vi "Write to Hardware.vi"(8 "error in":errorcluster, 9 "trigger values":dbl[](array[numeric]), 10 "values":dbl[](array[numeric]), 11 "tx execution unit":refnum<class "Tx Execution Unit.lvclass">) -> (0 "error out":errorcluster, 1 "trigger values out":dbl[](array[numeric]), 2 "values out":dbl[](array[numeric]), 3 "tx execution unit out":refnum<class "Tx Execution Unit.lvclass">)   [LabVIEW 2020, in "AIM MIL-STD-1553 Engine.lvlib" / "Implementation.lvlib" / "Tx Execution Unit.lvclass"]
uses:
  Tx Execution Unit.lvclass
  C:/dev/git/niveristand-aim-milStd1553-custom-device/Source/Custom Device Support/Engine/Implementation/Execution Unit/Execution Unit.lvclass
  Execution Unit/Execution Unit.lvclass/Execution Unit.ctl
  Tx Execution Unit.lvclass/Tx Execution Unit.ctl
  Shared/Message Definition.ctl
  Shared/Message Type.ctl
  Shared/Terminal Endpoint.ctl
  Shared/Address.ctl
  Shared/Parameter Definition.ctl
  Execution Unit/Read Module Reference.vi
  Read Transmitted Messages.vi
  Hardware API/AIM MIL-STD-1553 Hardware API.lvlib
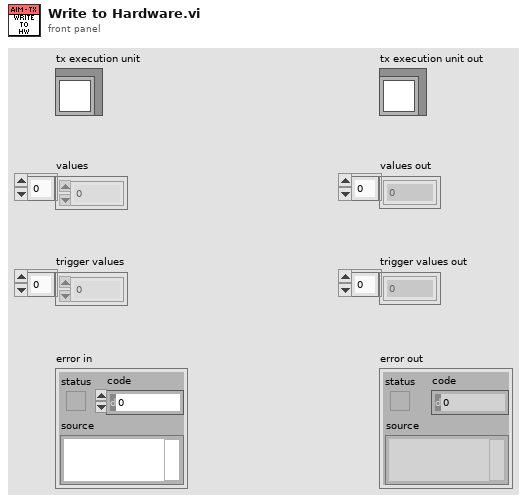
[diagram p1: front panel]
types:
  T1 = typedef "AIM MIL-STD-1553 Hardware API.lvlib/Module Reference.ctl" = u32
  T2 = typedef "AIM MIL-STD-1553 Engine.lvlib/Custom Device.lvlib/Compiled Message.ctl" = cluster{"Message Section Handle":T3, "First Parameter Index":i32, "Parameter Channel Handles":T3[], "Direction":T4, "Parameters":T5[], "Receiving RT Address":u8, "Receiving RT Sub-address":u8, "Transmitting RT Address":u8, "Transmitting RT Sub-address":u8, "Word Count":u8, "Buffer Type":enum16{"unknown", "BC Message Buffer", "RT Message Buffer"}, "Buffer ID":u16, "Terminal Type":enum16{"Bus Controller", "Remote Terminal"}, "Timestamp Enabled":bool, "Timestamp Channel Handle":T3}
  T3 = typedef "Custom Device API.lvlib/Custom Device Item Ref.ctl" = u64
  T4 = typedef "Direction.ctl" = enum16{"Rx", "Tx"}
  T5 = typedef "Parameter Definition.ctl" = cluster{"start index":i32, "size (bits)":i32, "encoding":enum16{"BNR", "BCD", "Discrete"}, "signed":bool, "multiplier":dbl, "offset":dbl}
  T6 = typedef "Message Definition.ctl" = cluster{"name":string, "message type":T7, "endpoint Tx":T8, "endpoint Rx":T8, "create timestamp channel":bool, "mode code":u16, "number of words":u16, "parameters":cluster{"name":string, "default value":dbl, "unit":string, "parameter definition":T5}[]}
  T7 = typedef "Message Type.ctl" = string
  T8 = typedef "Terminal Endpoint.ctl" = cluster{"terminal address":T9, "subaddress":T9}
  T9 = typedef "Address.ctl" = u16
  T10 = cluster{"name":string, "default value":dbl, "unit":string, "parameter definition":T5}
  T11 = enum16{"unknown", "BC Message Buffer", "RT Message Buffer"}
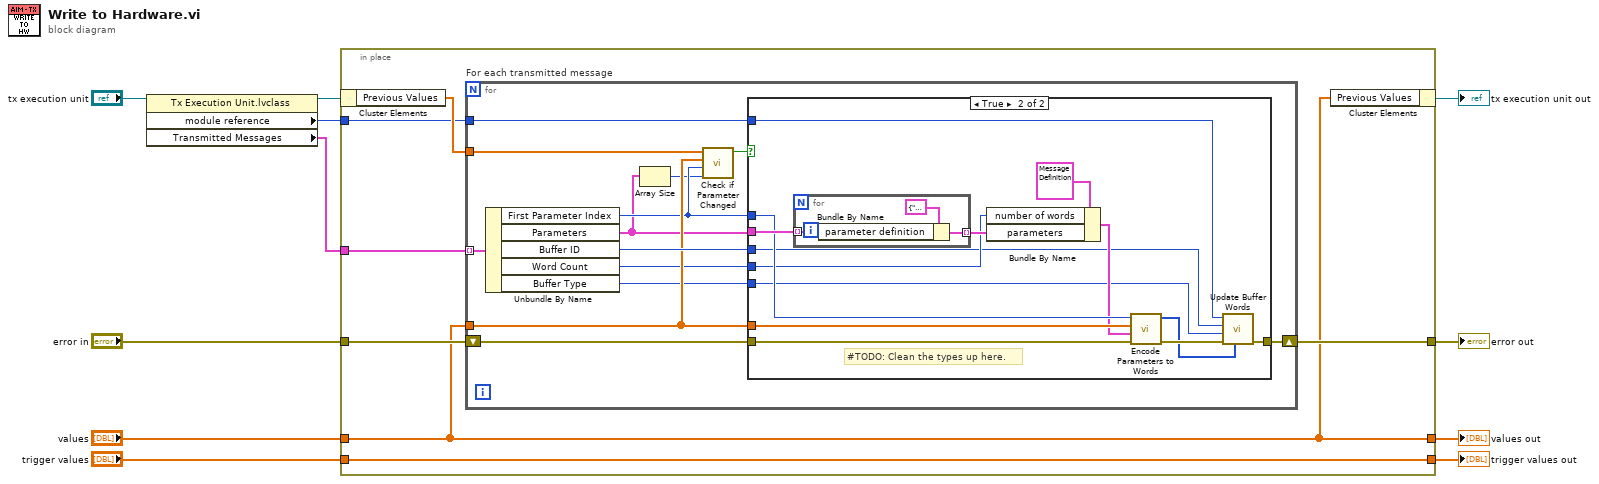
[diagram p0: block diagram]
diagram:
  n1 = property class="Tx Execution Unit.lvclass"(reference="tx execution unit") -> (reference out=w2:refnum<class "Tx Execution Unit.lvclass">, "module reference"=w3:T1, "Transmitted Messages"=w1:T2[])  [unwired: 1 in, 1 out]
  n2 = in-place {
    in-place-border: "values" -> [w15]
    in-place-border: "error in" -> [w18]
    in-place-border: [w17] -> w4
    in-place-border: [w16] -> w7
    in-place-border: "trigger values" -> [w16]
    in-place-border: [w15] -> w5
    in-place-border: w1 -> [w13]
    in-place-border: w3 -> [w12]
    n3 = in-place-cluster #1(w2) -> ("Previous Values"=w14:dbl[])
    n4 = for "For each transmitted message" {
      shift-right: [w31] -> w17
      shift-left: w18 -> [w30]
      tunnel: w14 -> [w28]
      tunnel: w15 -> [w25]
      tunnel: w13 -> [w29] mode=indexing
      tunnel: w12 -> [w19]
      n5 = Unbundle By Name(w29) -> ("First Parameter Index"=w24:i32, "Parameters"=w22:T5[], "Buffer ID"=w26:u16, "Word Count"=w21:u8, "Buffer Type"=w20:T11)
      n6 = Array Size(array=w22) -> (size(s)=w23:i32)
      n7 = call "Check if Parameter Changed.vi"("Number of Parameters"=w23, "First Parameter Index"=w24, "New Values"=w25, "Previous Values"=w28) -> ("parameter has changed"=w27:bool)  [unwired: 7 in]
      n8 = case shown="True" w27 {
        tunnel: [w32 w38] -> w31
        tunnel: w30 -> [w32 w46]
        tunnel: w26 -> [_ w36]
        tunnel: w25 -> [_ w45]
        tunnel: w24 -> [_ w41]
        tunnel: w22 -> [_ w43]
        tunnel: w21 -> [_ w40]
        tunnel: w20 -> [_ w35]
        tunnel: w19 -> [_ w37]
        frame False {
          # "None of the parameters have changed, so there is nothing to do.\n\nThe buffer is already up to date."
        }
        frame True {
          # "#TODO: Clean the types up here."
          n9 = for {
            tunnel: w43 -> [w48] mode=indexing
            tunnel: [w47] -> w42 mode=indexing
            n10 = Bundle By Name(cluster=T10 {"name"="", "default value"=0.0, "unit"="", "parameter definition"={"start index"=0, "size (bits)"=0, "encoding"=enum."BNR", "signed"=FALSE, "multiplier"=0.0, "offset"=0.0}} ("definition with default value"), "parameter definition"=w48) -> (w47:T10)
          }
          n11 = Bundle By Name(cluster=T6 {"name"="", "message type"="BC to RT", "endpoint Tx"={"terminal address"=0, "subaddress"=0}, "endpoint Rx"={"terminal address"=0, "subaddress"=0}, "create timestamp channel"=FALSE, "mode code"=0, "number of words"=0, "parameters"=[]} ("message"), "number of words"=w40, "parameters"=w42) -> (w39:T6)
          n12 = call "Encode Parameters to Words.vi"("error in"=w46, "message"=w39, "Values"=w45, "value index"=w41) -> ("error out"=w34:errorcluster, "data words"=w33:u16[])  [unwired: 6 in]
          n13 = call "Update Buffer Words.vi"("data word to write"=w33, "error in"=w34, "buffer type"=w35, "buffer id"=w36, "module handle"=w37) -> ("error out"=w38:errorcluster)  [unwired: 5 in, 1 out]
        }
      }
    }
    n14 = in-place-cluster #1("Previous Values"=w15) -> (→"tx execution unit out":refnum<class "Tx Execution Unit.lvclass">)
  }
  "error out" <- w4
  "values out" <- w5
  "trigger values out" <- w7
